vi "RESTful Configure VI Terminal Settings.vi"(6 "VI Section Heading":string, 7 "VI Name":string, 8 "error in":errorcluster, 9 "Terminal Info Summary":T1, 11 "Master Text In":string="#Terminals") -> (0 "error out":errorcluster, 3 "Master Text Out":string="#VIs")   [LabVIEW 2020]
doc: "This VI configures per-Terminal information for the webservices INI file."
uses:
  <vilib>/AppBuilder/Engine/RESTful INI Generator/RESTful VI Terminal Info Summary.ctl
  <resource>/Framework/Providers/Common/provcom_StringGlobals.vi
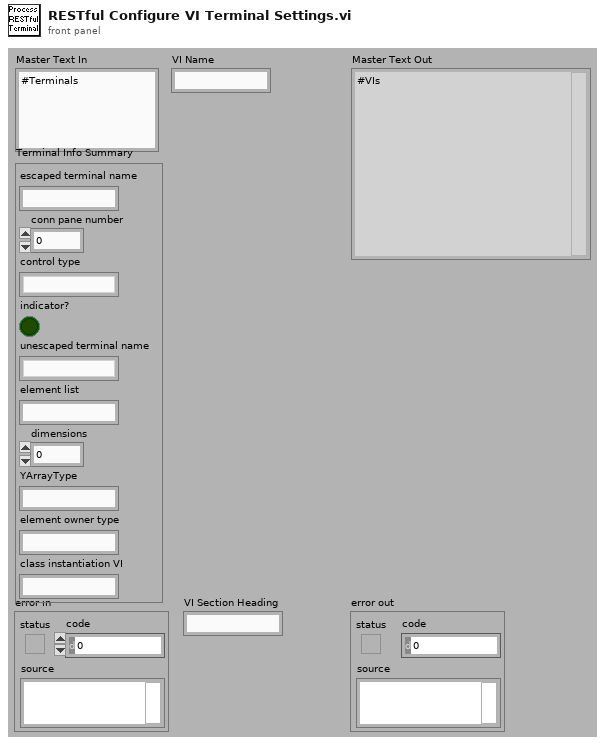
[diagram p1: front panel]
types:
  T1 = typedef "RESTful VI Terminal Info Summary.ctl" = cluster{"escaped terminal name":string, "conn pane number":i32, "control type":string, "indicator?":bool, "unescaped terminal name":string, "element list":string, "dimensions":u32, "YArrayType":string, "element owner type":string, "class instantiation VI":string}
  T2 = cluster{"main":string, "control ":string, "indicator":string}
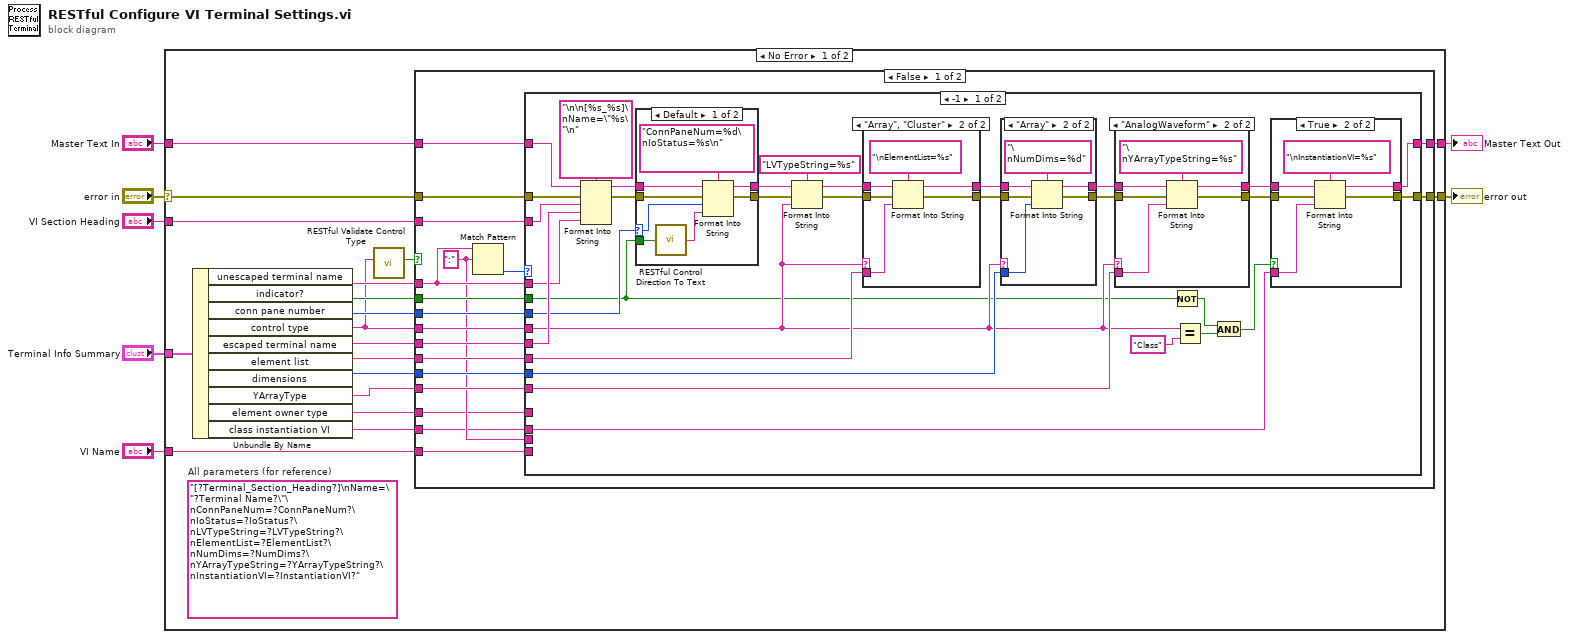
[diagram p0: block diagram]
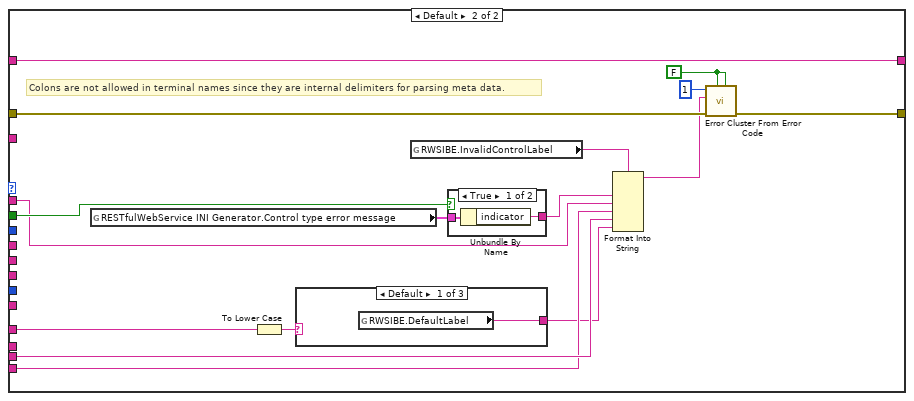
[diagram p7: hidden frame]
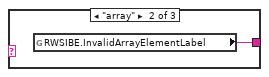
[diagram p8: hidden frame]
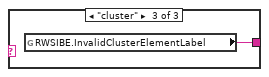
[diagram p9: hidden frame]
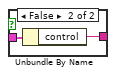
[diagram p10: hidden frame]
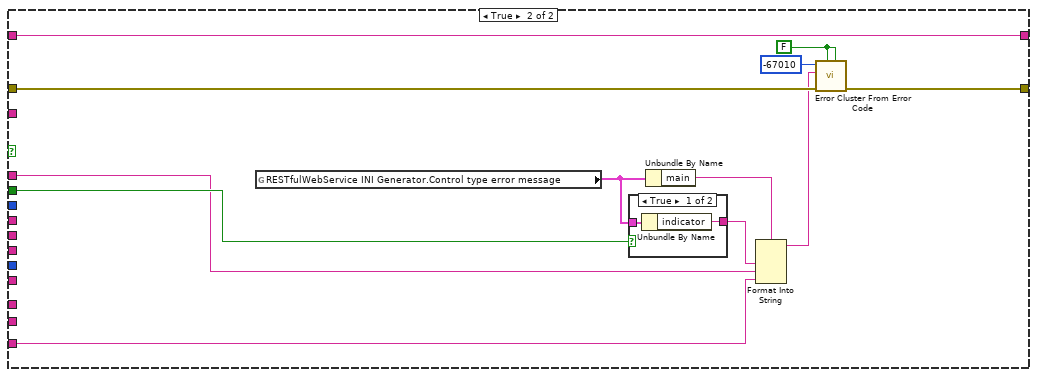
[diagram p11: hidden frame]
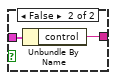
[diagram p12: hidden frame]
diagram:
  n1 = case shown="No Error" "error in" {
    selector: "error in" -> [w13 w157]
    tunnel: [w25 w157] -> w7
    tunnel: "Terminal Info Summary" -> [w12 _]
    tunnel: "VI Name" -> [w23 _]
    tunnel: "VI Section Heading" -> [w22 _]
    tunnel: "Master Text In" -> [w18 w158]
    tunnel: [w14 w158] -> w2
    frame No Error {
      (unwired) "[?Terminal_Section_Heading?]\nName=\"?Terminal Name?\"\nConnPaneNum=?ConnPaneNum?\nIoStatus=?IoStatus?\nLVTypeString=?LVTypeString?\nElementList=?ElementList?\nNumDims=?NumDims?\nYArrayTypeString=?YArrayTypeString?\nInstantiationVI=?InstantiationVI?"  # All parameters (for reference)
      n2 = Unbundle By Name(w12) -> ("unescaped terminal name"=w20:string, "indicator?"=w17:bool, "conn pane number"=w19:i32, "control type"=w15:string, "escaped terminal name"=w21:string, "element list"=w10:string, "dimensions"=w16:u32, "YArrayType"=w11:string, "element owner type"=w9:string, "class instantiation VI"=w8:string)
      n3 = call <vilib>:"RESTful Validate Control Type.vi"("Type String"=w15) -> ("Invalid RESTful Type?"=w24:bool)  [unwired: 10 out]
      n4 = case shown="False" w24 {
        tunnel: w18 -> [w41 w152]
        tunnel: [w40 w152] -> w14
        tunnel: w19 -> [w37 _]
        tunnel: w22 -> [w39 _]
        tunnel: [w42 w150] -> w25
        tunnel: w15 -> [w34 _]
        tunnel: w13 -> [w43 w149]
        tunnel: w21 -> [w38 _]
        tunnel: w17 -> [w36 w146]
        tunnel: w20 -> [w31 w144]
        tunnel: w23 -> [w28 w141]
        tunnel: w10 -> [w35 _]
        tunnel: w16 -> [w33 _]
        tunnel: w11 -> [w32 _]
        tunnel: w9 -> [w27 _]
        tunnel: w8 -> [w26 _]
        frame False {
          w29 = ":" ("regular expression")
          n5 = Match Pattern(string=w31, regular expression=w29) -> (offset past match=w30:i32)  [unwired: 1 in, 3 out]
          n6 = case shown="-1" w30 {
            tunnel: w43 -> [w68 w130]
            tunnel: [w53 w129] -> w42
            tunnel: w41 -> [w62 w133]
            tunnel: [w54 w133] -> w40
            tunnel: w39 -> [w61 _]
            tunnel: w38 -> [w60 _]
            tunnel: w31 -> [w59 w122]
            tunnel: w37 -> [w58 _]
            tunnel: w36 -> [w45 w125]
            tunnel: w35 -> [w57 _]
            tunnel: w34 -> [w49 _]
            tunnel: w33 -> [w56 _]
            tunnel: w32 -> [w55 _]
            tunnel: w29 -> [_ w124]
            tunnel: w28 -> [_ w121]
            tunnel: w27 -> [_ w119]
            tunnel: w26 -> [w50 _]
            frame -1 {
              n7 = Format Into String(format string="\n\n[%s_%s]\nName=\"%s\"\n", initial string=w62, error in=w68, w61, w60, w59) -> (resulting string=w70:string, error out=w67:errorcluster)
              n8 = case shown="Default" w58 {
                selector: w58 -> [w113 _]
                tunnel: w70 -> [w114 w117]
                tunnel: [w110 w117] -> w71
                tunnel: w45 -> [w111 _]
                tunnel: w67 -> [w109 w116]
                tunnel: [w108 w116] -> w66
                frame Default {
                  n9 = call <vilib>:"RESTful Control Direction To Text.vi"("Indicator?"=w111) -> ("Boolean Text"=w112:string)
                  n10 = Format Into String(format string="ConnPaneNum=%d\nIoStatus=%s\n", initial string=w114, error in=w109, w113, w112) -> (resulting string=w110:string, error out=w108:errorcluster)
                }
                frame -1 {
                }
              }
              n11 = Format Into String(format string="LVTypeString=%s", initial string=w71, error in=w66, w49) -> (resulting string=w73:string, error out=w65:errorcluster)
              n12 = case shown="\"Array\", \"Cluster\"" w49 {
                tunnel: w73 -> [w101 w106]
                tunnel: w57 -> [_ w105]
                tunnel: [w101 w104] -> w74
                tunnel: w65 -> [w100 w103]
                tunnel: [w100 w102] -> w64
                frame Default {
                }
                frame "Array", "Cluster" {
                  n13 = Format Into String(format string="\nElementList=%s", initial string=w106, error in=w103, w105) -> (resulting string=w104:string, error out=w102:errorcluster)
                }
              }
              n14 = case shown="\"Array\"" w49 {
                tunnel: w74 -> [w93 w98]
                tunnel: w56 -> [_ w97]
                tunnel: [w93 w96] -> w75
                tunnel: w64 -> [w92 w95]
                tunnel: [w92 w94] -> w63
                frame Default {
                }
                frame "Array" {
                  n15 = Format Into String(format string="\nNumDims=%d", initial string=w98, error in=w95, w97) -> (resulting string=w96:string, error out=w94:errorcluster)
                }
              }
              n16 = case shown="\"AnalogWaveform\"" w49 {
                tunnel: w75 -> [w85 w90]
                tunnel: w55 -> [_ w89]
                tunnel: [w85 w88] -> w52
                tunnel: w63 -> [w84 w87]
                tunnel: [w84 w86] -> w51
                frame Default {
                }
                frame "AnalogWaveform" {
                  n17 = Format Into String(format string="\nYArrayTypeString=%s", initial string=w90, error in=w87, w89) -> (resulting string=w88:string, error out=w86:errorcluster)
                }
              }
              n18 = Not(x=w45) -> (.not. x?=w46:bool)
              n19 = Equal?(x=w49, y="Class") -> (x = y?=w47:bool)
              n20 = And(x=w46, y=w47) -> (x .and. y?=w44:bool)
              n21 = case shown="True" w44 {
                tunnel: w52 -> [w77 w82]
                tunnel: w50 -> [_ w81]
                tunnel: [w77 w80] -> w54
                tunnel: w51 -> [w76 w79]
                tunnel: [w76 w78] -> w53
                frame False {
                }
                frame True {
                  n22 = Format Into String(format string="\nInstantiationVI=%s", initial string=w82, error in=w79, w81) -> (resulting string=w80:string, error out=w78:errorcluster)
                }
              }
            }
            frame Default {
              w131 = FALSE ("is warning? (False)")
              # "Colons are not allowed in terminal names since they are internal delimiters for parsing meta data."
              n23 = global read "provcom_StringGlobals.vi" "RESTfulWebService INI Generator.Control type error message"() -> (w126:T2)
              n24 = To Lower Case(string=w119) -> (all lower case string=w118:string)
              n25 = case shown="Default" w118 {
                tunnel: [w134 w135 w136] -> w120
                frame Default {
                  n26 = global read "provcom_StringGlobals.vi" "RWSIBE.DefaultLabel"() -> (w134:string)
                }
                frame "array" {
                  n27 = global read "provcom_StringGlobals.vi" "RWSIBE.InvalidArrayElementLabel"() -> (w135:string)
                }
                frame "cluster" {
                  n28 = global read "provcom_StringGlobals.vi" "RWSIBE.InvalidClusterElementLabel"() -> (w136:string)
                }
              }
              n29 = global read "provcom_StringGlobals.vi" "RWSIBE.InvalidControlLabel"() -> (w128:string)
              n30 = case shown="True" w125 {
                tunnel: w126 -> [w138 w140]
                tunnel: [w137 w139] -> w123
                frame True {
                  n31 = Unbundle By Name(w138) -> ("indicator"=w137:string)
                }
                frame False {
                  n32 = Unbundle By Name(w140) -> ("control"=w139:string)
                }
              }
              n33 = Format Into String(format string=w128, w123, w122, w121, w124, w120) -> (resulting string=w127:string)  [unwired: 2 in, 1 out]
              n34 = call <vilib>:"Error Cluster From Error Code.vi"("is warning? (False)"=w131, "show call chain? (False)"=w131, "error in (no error)"=w130, "error message (\"\")"=w127, "error code (0)"=1) -> ("error out"=w129:errorcluster)  [unwired: 4 out]
            }
          }
        }
        frame True {
          w142 = FALSE ("is warning? (False)")
          n35 = global read "provcom_StringGlobals.vi" "RESTfulWebService INI Generator.Control type error message"() -> (w147:T2)
          n36 = case shown="True" w146 {
            tunnel: w147 -> [w154 w156]
            tunnel: [w153 w155] -> w145
            frame True {
              n37 = Unbundle By Name(w154) -> ("indicator"=w153:string)
            }
            frame False {
              n38 = Unbundle By Name(w156) -> ("control"=w155:string)
            }
          }
          n39 = Unbundle By Name(w147) -> ("main"=w148:string)
          n40 = Format Into String(format string=w148, w145, w144, w141) -> (resulting string=w143:string)  [unwired: 2 in, 1 out]
          n41 = call <vilib>:"Error Cluster From Error Code.vi"("is warning? (False)"=w142, "show call chain? (False)"=w142, "error in (no error)"=w149, "error message (\"\")"=w143, "error code (0)"=-67010) -> ("error out"=w150:errorcluster)  [unwired: 4 out]
        }
      }
    }
    frame Error {
    }
  }
  "error out" <- w7
  "Master Text Out" <- w2
